vi "CCD 多线程尝试.vi"(8 "error in (no error)":errorcluster caption="错误输入（无错误）", 9 "CCD stop":bool) -> (0 "error out":errorcluster caption="错误输出", 2 "Frame Rate":dbl, 3 "camera window":T1(plugin-control))   [LabVIEW 2017]
doc: "该模板用于创建子VI。"
uses:
  <vilib>/vision/driver/NI_Vision_Acquisition_Software.lvlib
panel:
  out "processed FPS":dbl
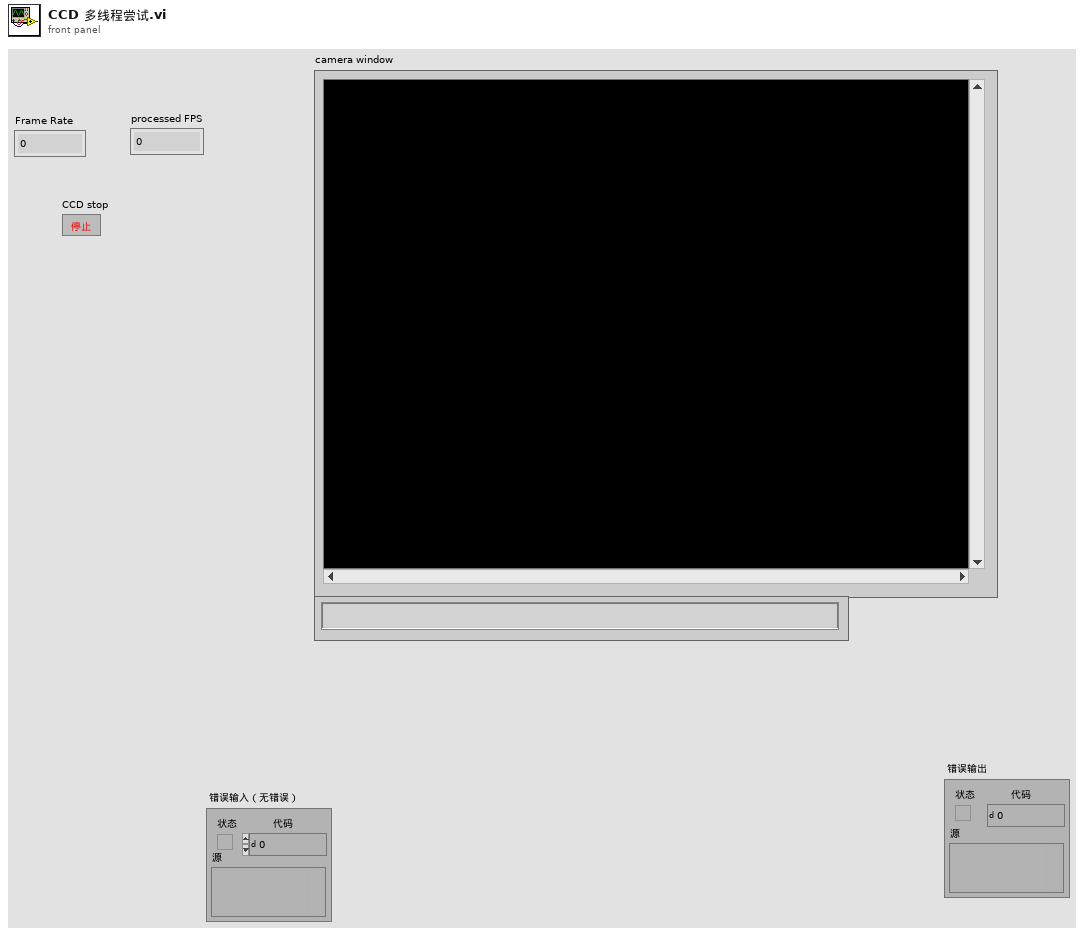
[diagram p1: front panel]
types:
  T1 = typedef "IMAQ Image.ctl" = refnum<image>
  T2 = typedef "IMAQdx.ctl" = refnum<k21>
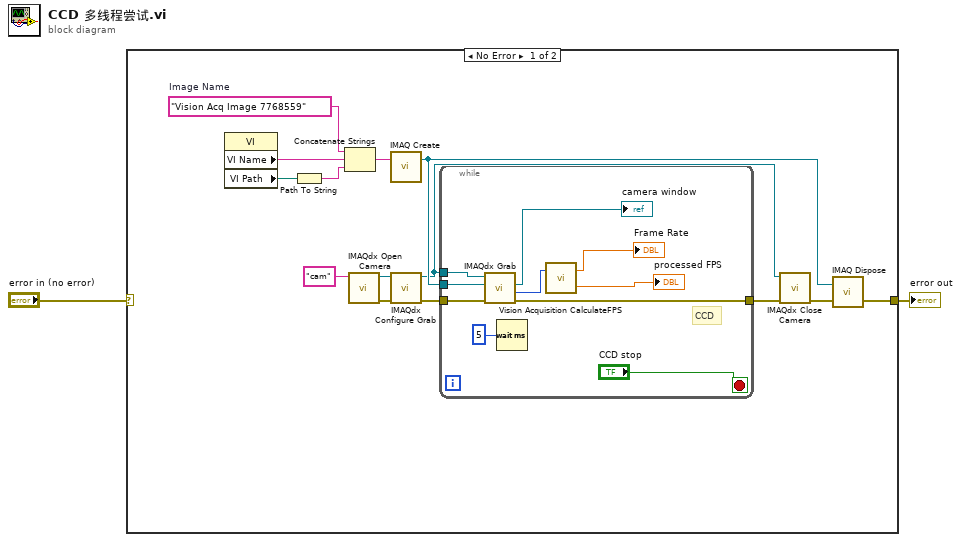
[diagram p0: block diagram]
diagram:
  n1 = case shown="No Error" "error in (no error)" {
    selector: "error in (no error)" -> [_ w27]
    tunnel: [w3 w27] -> w1
    frame No Error {
      w11 = "Vision Acq Image 7768559"  # Image Name
      n2 = property class="VI"() -> ("VI Name"=w14:string, "VI Path"=w15:path)  [unwired: 2 in, 2 out]
      n3 = Path To String(path=w15) -> (string=w13:string)
      n4 = Concatenate Strings(w11, w14, w13) -> (w12:string)
      n5 = call <vilib>:"IMAQdx Open Camera.vi"("Session In"="cam" ("Interface Name")) -> ("error out"=w10:errorcluster, "Session Out"=w9:T2)  [unwired: 2 in, 7 out]
      n6 = call "IMAQ Create"("Image Name"=w12) -> ("New Image"=w5:T1)  [unwired: 3 in, 2 out]
      n7 = call <vilib>:"IMAQdx Configure Grab.vi"("error in"=w10, "Session In"=w9) -> ("error out"=w8:errorcluster, "Session Out"=w4:T2)  [unwired: 8 out]
      n8 = while {
        tunnel: w4 -> [w25]
        tunnel: w5 -> [w24]
        tunnel: w8 -> [w22]
        tunnel: [w23] -> w6
        stop <- "CCD stop" stop-if-true
        # "CCD"
        n9 = call <vilib>:"IMAQdx Grab.vi"("error in"=w22, "Image In"=w24, "Session In"=w25) -> ("error out"=w23:errorcluster, "Buffer Number Out"=w26:u32, "Image Out"=→"camera window":T1)  [unwired: 1 in, 5 out]
        n10 = Wait (ms)(milliseconds to wait=u32 5 ("等待时间（毫秒）")) -> ()  [unwired: 1 out]
        n11 = call <vilib>:"Vision Acquisition CalculateFPS.vi"("buffer number"=w26) -> ("processed FPS"=→"processed FPS":dbl, "acquired FPS"=→"Frame Rate":dbl)  [unwired: 1 out]
      }
      n12 = call <vilib>:"IMAQdx Close Camera.vi"("error in"=w6, "Session In"=w4) -> ("error out"=w7:errorcluster)  [unwired: 9 out]
      n13 = call "IMAQ Dispose"("Image"=w5, "error in (no error)"=w7) -> ("error out"=w3:errorcluster)  [unwired: 4 in]
    }
    frame Error {
    }
  }
  "error out" <- w1
